vi "Get Slot.vi"(8 "error in":errorcluster, 11 "slot ref in":T1 format="%.0x") -> (0 "error out":errorcluster, 2 "module":refnum<class "Module.lvclass">, 3 "slot ref out":T1 format="%.0x", 4 "empty":bool)   [LabVIEW 2017, in "Scan Engine Scripting.lvlib"]
uses:
  Scan Engine Scripting.lvlib
  <vilib>/NI Veristand/Custom Device API/Custom Device Item Ref.ctl
  Modules/Module/Module.lvclass
  Modules.lvlibp/SD Module/SD Module.lvclass
  C:/dev/niveristand-scan-engine-ethercat-custom-device/Custom Device Source/Modules.lvlibp/RSI Module/RSI Module.lvclass
  Globals/Error Strings.vi
  Modules.lvlibp/RSI Module/RSI Module.lvclass
  Scan Engine Custom Device.lvlib
  <vilib>/NI Veristand/Custom Device API/Custom Device API.lvlib
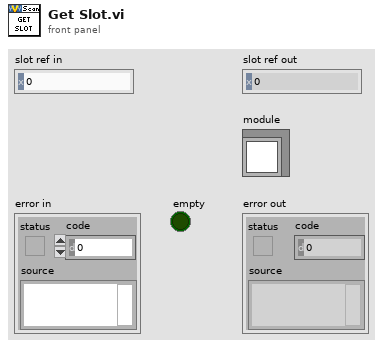
[diagram p1: front panel]
types:
  T1 = typedef "Custom Device API.lvlib/Custom Device Item Ref.ctl" = u64
  T2 = typedef "Modules.lvlibp/Custom Device API.lvlib/Custom Device Item Ref.ctl" = u64
  T3 = typedef "Modules.lvlibp/RSI Module.lvclass/Module Models.ctl" = enum16{"Empty", "NI 9201", "NI 9203", "NI 9205", "NI 9206", "NI 9207", "NI 9208", "NI 9209", "NI 9210", "NI 9211", "NI 9212", "NI 9213", "NI 9214", "NI 9215", "NI 9216", "NI 9217", "NI 9219", "NI 9220", "NI 9221", "NI 9222", "NI 9223", "NI 9224", "NI 9225", "NI 9226", "NI 9227", "NI 9228", "NI 9229", "NI 9233", "NI 9234", "NI 9235", "NI 9236", "NI 9237", "NI 9239", "NI 9242", "NI 9244", "NI 9253", "NI 9263", "NI 9264", "NI 9265", "NI 9266", "NI 9269", "NI 9344", "NI 9350", "NI 9375", "NI 9401", "NI 9402", "NI 9403", "NI 9411", "NI 9421", "NI 9422", "NI 9423", "NI 9425", "NI 9426", "NI 9435", "NI 9436", "NI 9437", "NI 9472", "NI 9474", "NI 9475", "NI 9476", "NI 9477", "NI 9478", "NI 9481", "NI 9482", "NI 9485"}
  T4 = typedef "Modules.lvlibp/RSI Module.lvclass/Channels.ctl" = cluster{"# Input Channels":i32, "# Output Channels":i32, "Channel Type":T5, "Units":string}
  T5 = typedef "Modules.lvlibp/RSI Module.lvclass/Channel Type.ctl" = enum16{"Analog", "Digital"}
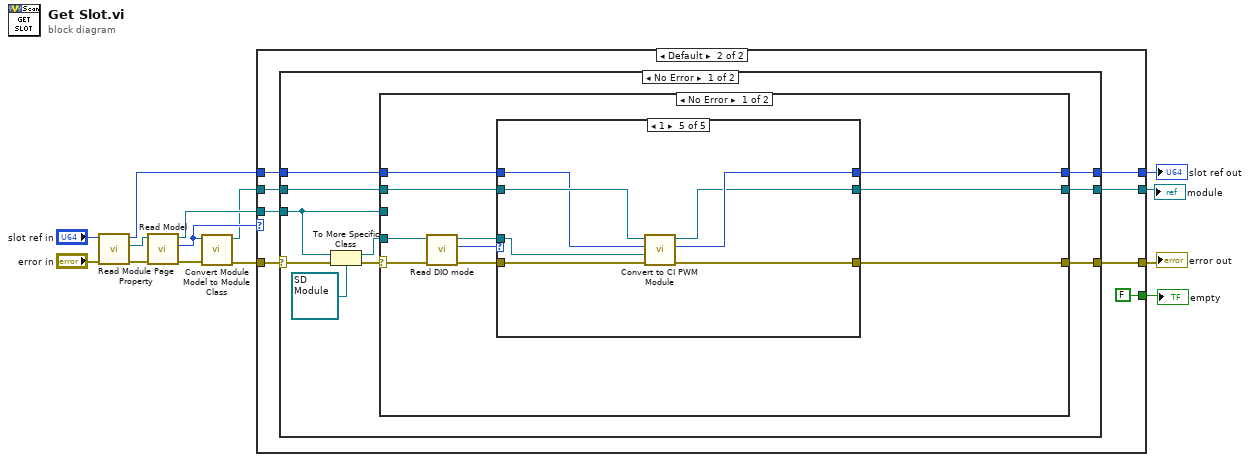
[diagram p0: block diagram]
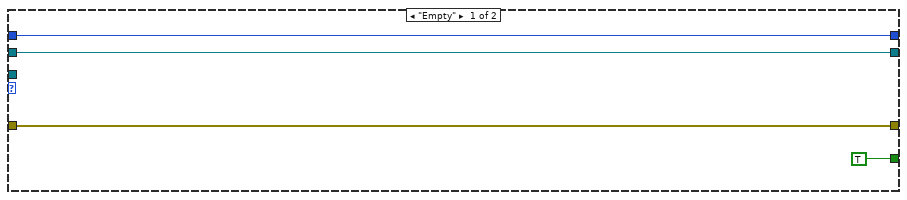
[diagram p2: hidden frame]
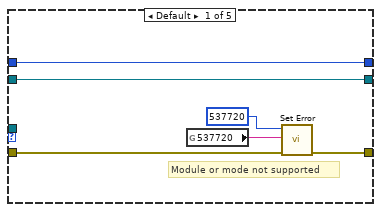
[diagram p3: hidden frame]
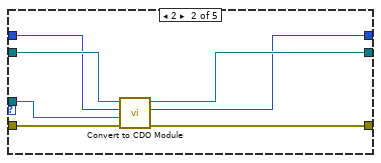
[diagram p4: hidden frame]
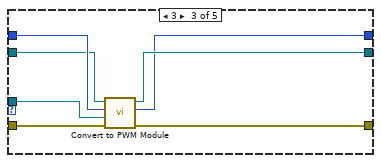
[diagram p5: hidden frame]
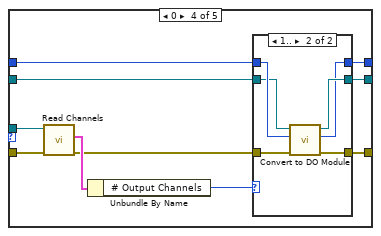
[diagram p6: hidden frame]
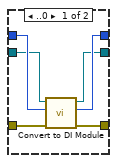
[diagram p7: hidden frame]
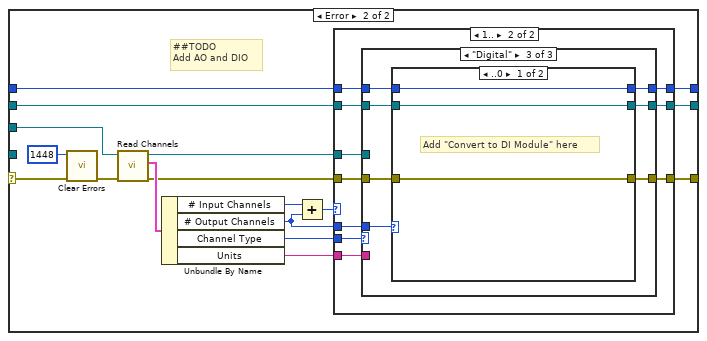
[diagram p8: hidden frame]
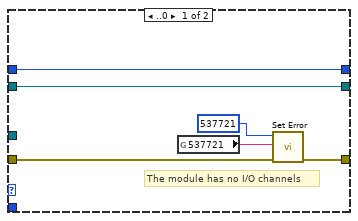
[diagram p9: hidden frame]
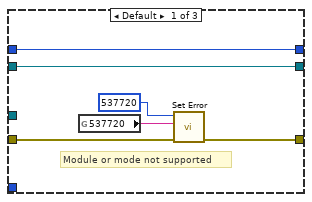
[diagram p10: hidden frame]
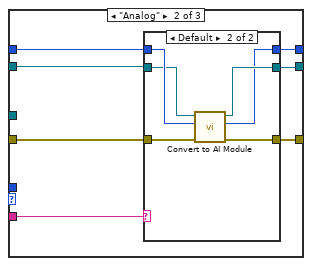
[diagram p11: hidden frame]
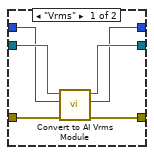
[diagram p12: hidden frame]
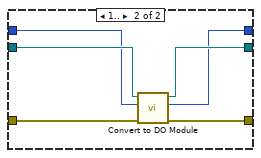
[diagram p13: hidden frame]
diagram:
  n1 = call "Read Module Page Property.vi"("error in (no error)"="error in", "Node Ptr In"="slot ref in") -> ("error out"=w6:errorcluster, "RSI Module"=w10:refnum<class "RSI Module.lvclass">, "Node Ptr Out"=w7:T2)  [unwired: 7 in]
  n2 = call "Read Model.vi"("error in (no error)"=w6, "RSI Module in"=w10) -> ("error out"=w5:errorcluster, "Model"=w3:T3, "RSI Module out"=w8:refnum<class "RSI Module.lvclass">)  [unwired: 7 in]
  n3 = call "Convert Module Model to Module Class.vi"("error in"=w5, "module model"=w3) -> ("error out"=w4:errorcluster, "module"=w2:refnum<class "Module.lvclass">)  [unwired: 8 in]
  n4 = case shown="Default" w3 {
    tunnel: [w18 w26] -> w14
    tunnel: [w16 w25] -> w13
    tunnel: [w17 w24] -> w9
    tunnel: w8 -> [_ w23]
    tunnel: w7 -> [w16 w22]
    tunnel: w4 -> [w18 w20]
    tunnel: w2 -> [w17 w21]
    tunnel: [TRUE ("empty") FALSE ("empty")] -> w1
    frame "Empty" {
    }
    frame Default {
      n5 = case shown="No Error" w20 {
        selector: w20 -> [w28 w172]
        tunnel: [w36 w172] -> w26
        tunnel: [w35 w171] -> w25
        tunnel: [w34 w170] -> w24
        tunnel: w23 -> [w27 _]
        tunnel: w21 -> [w33 w170]
        tunnel: w22 -> [w32 w171]
        frame No Error {
          n6 = To More Specific Class(target class=refnum<class "SD Module.lvclass"> refnum ("Modules.lvlibp:SD Module.lvclass"), reference=w27, error in=w28) -> (specific class reference=w30:refnum<class "SD Module.lvclass">, error out=w29:errorcluster)
          n7 = case shown="No Error" w29 {
            selector: w29 -> [w40 w111]
            tunnel: [w46 w101] -> w36
            tunnel: [w39 w104] -> w35
            tunnel: [w45 w102] -> w34
            tunnel: w33 -> [w44 w103]
            tunnel: w32 -> [w38 w105]
            tunnel: w30 -> [w41 _]
            tunnel: w27 -> [_ w100]
            frame No Error {
              n8 = call "Read DIO mode.vi"("error in (no error)"=w40, "SD Module in"=w41) -> ("error out"=w37:errorcluster, "DIO mode"=w43:u32, "SD Module out"=w42:refnum<class "SD Module.lvclass">)  [unwired: 7 in]
              n9 = case shown="1" w43 {
                tunnel: [w48 w58 w61 w73 w91] -> w46
                tunnel: w42 -> [_ w55 w65 w70 w89]
                tunnel: w37 -> [w49 w56 w66 w71 w92]
                tunnel: [w51 w57 w62 w74 w90] -> w45
                tunnel: w44 -> [w51 w59 w63 w75 w95]
                tunnel: w38 -> [w52 w54 w64 w76 w94]
                tunnel: [w52 w53 w60 w72 w93] -> w39
                frame Default {
                  # "Module or mode not supported"
                  n10 = global read "Error Strings.vi" "537720"() -> (w47:string)
                  n11 = call "Set Error.vi"("error in (no error)"=w49, "Message"=w47, "Code"=537720) -> ("error out"=w48:errorcluster)  [unwired: 8 in]
                }
                frame 2 {
                  n12 = call "Convert to CDO Module.vi"("error in"=w56, "SD Module in"=w55, "slot ref in"=w54, "module in"=w59) -> ("error out"=w58:errorcluster, "slot ref out"=w53:T1, "module out"=w57:refnum<class "Module.lvclass">)  [unwired: 4 in, 1 out]
                }
                frame 3 {
                  n13 = call "Convert to PWM Module.vi"("error in"=w66, "SD Module in"=w65, "slot ref in"=w64, "module in"=w63) -> ("error out"=w61:errorcluster, "slot ref out"=w60:T1, "module out"=w62:refnum<class "Module.lvclass">)  [unwired: 4 in, 1 out]
                }
                frame 0 {
                  n14 = call "Read Channels.vi"("error in (no error)"=w71, "RSI Module in"=w70) -> ("error out"=w67:errorcluster, "Channels"=w69:T4)  [unwired: 7 in, 1 out]
                  n15 = Unbundle By Name(w69) -> ("# Output Channels"=w68:i32)
                  n16 = case shown="1.." w68 {
                    tunnel: w76 -> [w80 w88]
                    tunnel: w75 -> [w78 w87]
                    tunnel: [w77 w86] -> w74
                    tunnel: [w81 w85] -> w73
                    tunnel: [w79 w84] -> w72
                    tunnel: w67 -> [w82 w83]
                    frame ..0 {
                      n17 = call "Convert to DI Module.vi"("error in"=w82, "slot ref in"=w80, "module in"=w78) -> ("error out"=w81:errorcluster, "slot ref out"=w79:T1, "module out"=w77:refnum<class "Module.lvclass">)  [unwired: 6 in]
                    }
                    frame 1.. {
                      n18 = call "Convert to DO Module.vi"("error in"=w83, "slot ref in"=w88, "module in"=w87) -> ("error out"=w85:errorcluster, "slot ref out"=w84:T1, "module out"=w86:refnum<class "Module.lvclass">)  [unwired: 6 in]
                    }
                  }
                }
                frame 1 {
                  n19 = call "Convert to CI PWM Module.vi"("error in"=w92, "SD Module in"=w89, "slot ref in"=w94, "module in"=w95) -> ("error out"=w91:errorcluster, "slot ref out"=w93:T1, "module out"=w90:refnum<class "Module.lvclass">)  [unwired: 4 in, 1 out]
                }
              }
            }
            frame Error {
              # "##TODO\nAdd AO and DIO"
              n20 = call <vilib>:"Clear Errors.vi"("error in (no error)"=w111, "specific error code to clear (0: all)"=1448) -> ("error out"=w106:errorcluster)  [unwired: 4 in, 1 out]
              n21 = call "Read Channels.vi"("error in (no error)"=w106, "RSI Module in"=w100) -> ("error out"=w108:errorcluster, "Channels"=w110:T4, "RSI Module out"=w109:refnum<class "RSI Module.lvclass">)  [unwired: 7 in]
              n22 = Unbundle By Name(w110) -> ("# Input Channels"=w99:i32, "# Output Channels"=w96:i32, "Channel Type"=w97:T5, "Units"=w107:string)
              n23 = Add(x=w99, y=w96) -> (x+y=w98:i32)
              n24 = case shown="1.." w98 {
                tunnel: w109 -> [_ w128]
                tunnel: w108 -> [w114 w127]
                tunnel: w107 -> [_ w126]
                tunnel: w105 -> [w118 w125]
                tunnel: [w118 w124] -> w104
                tunnel: w103 -> [w117 w123]
                tunnel: [w117 w122] -> w102
                tunnel: [w113 w121] -> w101
                tunnel: w97 -> [_ w120]
                tunnel: w96 -> [_ w119]
                frame ..0 {
                  # "The module has no I/O channels"
                  n25 = global read "Error Strings.vi" "537721"() -> (w116:string)
                  n26 = call "Set Error.vi"("error in (no error)"=w114, "Message"=w116, "Code"=537721) -> ("error out"=w113:errorcluster)  [unwired: 8 in]
                }
                frame 1.. {
                  n27 = case shown="\"Digital\"" w120 {
                    tunnel: w128 -> [_ _ _]
                    tunnel: w127 -> [w131 w138 w154]
                    tunnel: w123 -> [w134 w139 w156]
                    tunnel: w125 -> [w133 w140 w158]
                    tunnel: w126 -> [_ w141 _]
                    tunnel: [w130 w137 w155] -> w121
                    tunnel: [w134 w136 w157] -> w122
                    tunnel: [w133 w135 w159] -> w124
                    tunnel: w119 -> [_ _ w160]
                    frame Default {
                      # "Module or mode not supported"
                      n28 = global read "Error Strings.vi" "537720"() -> (w132:string)
                      n29 = call "Set Error.vi"("error in (no error)"=w131, "Message"=w132, "Code"=537720) -> ("error out"=w130:errorcluster)  [unwired: 8 in]
                    }
                    frame "Analog" {
                      n30 = case shown="Default" w141 {
                        tunnel: w140 -> [w146 w152]
                        tunnel: w139 -> [w147 w151]
                        tunnel: w138 -> [w145 w153]
                        tunnel: [w144 w148] -> w137
                        tunnel: [w143 w150] -> w136
                        tunnel: [w142 w149] -> w135
                        frame "Vrms" {
                          n31 = call "Convert to AI Vrms Module.vi"("error in"=w145, "slot ref in"=w146, "module in"=w147) -> ("error out"=w144:errorcluster, "slot ref out"=w142:T1, "module out"=w143:refnum<class "Module.lvclass">)  [unwired: 6 in]
                        }
                        frame Default {
                          n32 = call "Convert to AI Module.vi"("error in"=w153, "slot ref in"=w152, "module in"=w151) -> ("error out"=w148:errorcluster, "slot ref out"=w149:T1, "module out"=w150:refnum<class "Module.lvclass">)  [unwired: 6 in]
                        }
                      }
                    }
                    frame "Digital" {
                      n33 = case shown="..0" w160 {
                        tunnel: [w163 w165] -> w159
                        tunnel: w158 -> [w163 w168]
                        tunnel: [w162 w166] -> w157
                        tunnel: w156 -> [w162 w169]
                        tunnel: [w161 w164] -> w155
                        tunnel: w154 -> [w161 w167]
                        frame ..0 {
                          # "Add \"Convert to DI Module\" here"
                        }
                        frame 1.. {
                          n34 = call "Convert to DO Module.vi"("error in"=w167, "slot ref in"=w168, "module in"=w169) -> ("error out"=w164:errorcluster, "slot ref out"=w165:T1, "module out"=w166:refnum<class "Module.lvclass">)  [unwired: 6 in]
                        }
                      }
                    }
                  }
                }
              }
            }
          }
        }
        frame Error {
        }
      }
    }
  }
  "error out" <- w14
  "slot ref out" <- w13
  "module" <- w9
  "empty" <- w1
